vi "Joint Manipulator Inertia (Point).vi"(8 "error in (no error)":errorcluster, 10 "joint positions":dbl[](array[numeric]), 11 "serial arm in":refnum<class "NI_Robotics_Serial Robot Arm.lvclass">) -> (0 "error out":errorcluster, 2 "inertia matrix":T1, 3 "serial arm out":refnum<class "NI_Robotics_Serial Robot Arm.lvclass">)   [LabVIEW 2017, in "NI_Kinematics.lvlib"]
doc: "Calculates a matrix that represents the kinetic energy of the end effector of a robotic arm in joint space. Wire data to the <B>joint positions</B> input to determine the polymorphic instance to use or manually select the instance. \n\n<B>.m file:</B> inertia"
uses:
  <vilib>/robotics/Kinematics/NI_Kinematics.lvlib
  <vilib>/robotics/Kinematics/Robot/NI_Robotics_Serial Robot Arm.lvclass
  <vilib>/Analysis/Matrix/Datatypes/RealMatrix.ctl
  <vilib>/Analysis/baseanly.llb/Real Outer Product.vi
  <vilib>/robotics/Kinematics/dyn/Inverse Dynamics (Trajectory).vi
  <vilib>/Analysis/7linalg.llb/Create Special Real Matrix.vi
  <vilib>/Analysis/NI_AALBase.lvlib
  <vilib>/Analysis/Matrix/NI_Matrix.lvlib
  <vilib>/Analysis/NI_AALPro.lvlib
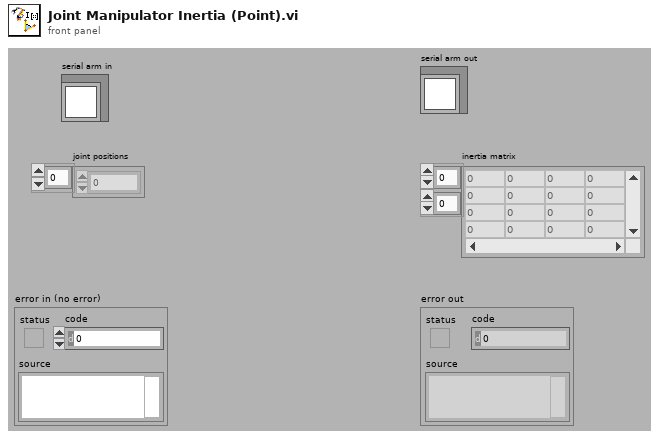
[diagram p1: front panel]
types:
  T1 = typedef "NI_Matrix.lvlib/RealMatrix.ctl" = dbl[][]
  T2 = enum32{"Identity", "Diagonal", "Toepliz", "Vandermonde", "Companion"}
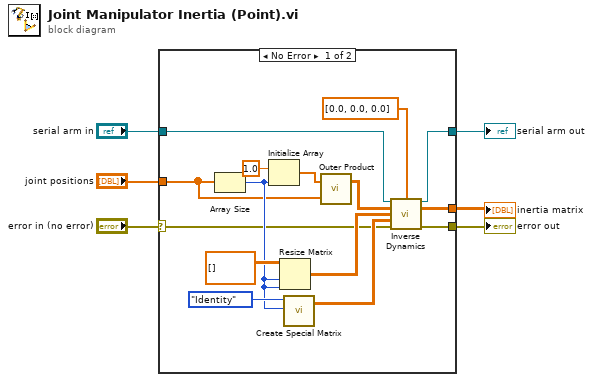
[diagram p0: block diagram]
diagram:
  n1 = case shown="No Error" "error in (no error)" {
    selector: "error in (no error)" -> [w7 w22]
    tunnel: [w12 w23] -> w6
    tunnel: "serial arm in" -> [w11 w23]
    tunnel: "joint positions" -> [w10 _]
    tunnel: [w9 _] -> w3
    tunnel: [w8 w22] -> w2
    frame No Error {
      n2 = Array Size(array=w10) -> (size(s)=w13:i32)
      n3 = Initialize Array(1.0 ("element"), w13) -> (w20:dbl[])
      n4 = Resize Matrix(1:w13, 2:w13, 4:T1 [] ("matrix")) -> (0:w17:T1)
      n5 = call-poly <vilib>:"Create Special Matrix.vi"("matrix type"=T2."Identity", "matrix size"=w13) -> ("Special Matrix"=w15:T1)  [unwired: 3 in, 1 out]
      n6 = call-poly <vilib>:"Outer Product.vi"("Y Vector"=w10, "X Vector"=w20) -> ("Outer Product"=w19:T1)  [unwired: 1 out]
      n7 = call-poly <vilib>:"Inverse Dynamics.vi"("serial arm in"=w11, "gravity"=dbl[] [0.0, 0.0, 0.0], "joint position trajectory"=w19, "joint velocity trajectory"=w17, "joint acceleration trajectory"=w15, "error in (no error)"=w7) -> ("serial arm out"=w12:refnum<class "NI_Robotics_Serial Robot Arm.lvclass">, "required torque trajectory"=w9:dbl[][], "error out"=w8:errorcluster)  [unwired: 7 in]
    }
    frame Error {
    }
  }
  "serial arm out" <- w6
  "inertia matrix" <- w3
  "error out" <- w2
